vi "openCV_py.vi"() -> (2 "Move by":dbl[](array[numeric]))   [LabVIEW 2020]
panel:
  out "error out":errorcluster
  in  "error in (no error)":errorcluster
  in  "python module path":path=path "C:/Users/HEP/Documents/GitHub/UCSB-Gantry-HEP/Main VIs/LV_CV/py_cv.py"
  in  "python function name":string="get_new_loc"
  in  "Python version":string="3.6"
  out "PY time":dbl=1508.0
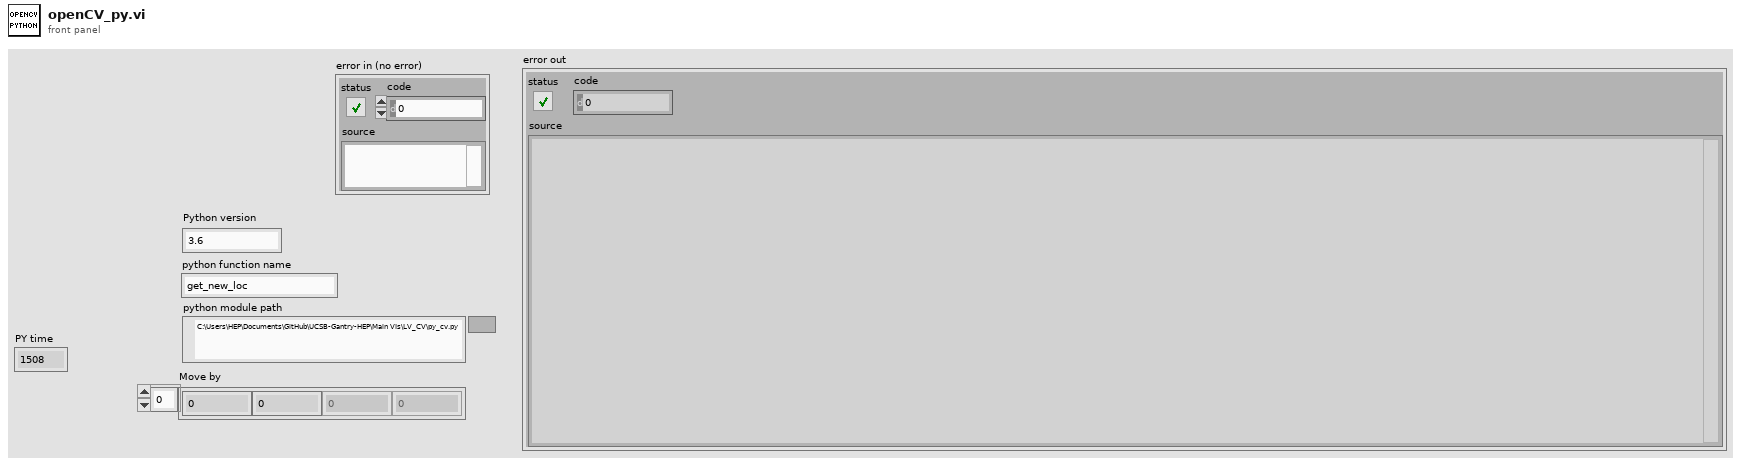
[diagram p1: front panel]
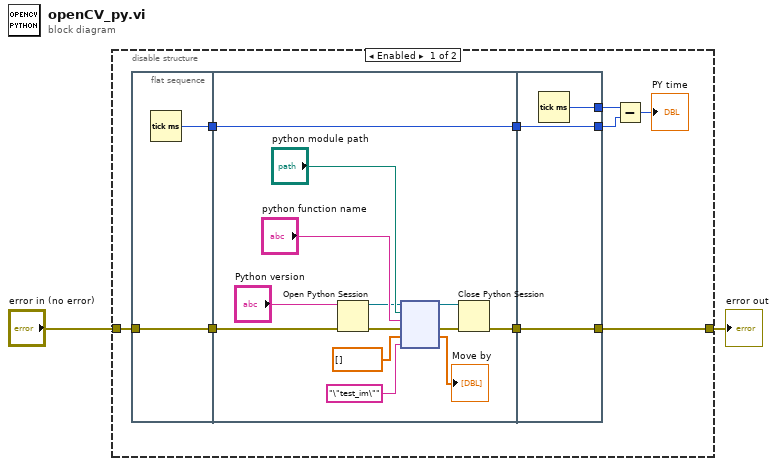
[diagram p0: block diagram]
diagram:
  n1 = disable-structure shown="Enabled" {
    disable-tunnel: "error in (no error)" -> [w7 _]
    disable-tunnel: [w6 _] -> w2
    frame Enabled {
      n2 = flat-sequence {
        tunnel: w7 -> [w13]
        tunnel: [w13] -> w11
        tunnel: [w12] -> w10
        tunnel: w11 -> [w21]
        tunnel: [w18] -> w9
        tunnel: [w17] -> w8
        tunnel: w10 -> [w17]
        tunnel: [w29] -> w6
        tunnel: w9 -> [w29]
        tunnel: [w28] -> w5
        tunnel: [w27] -> w4
        tunnel: w8 -> [w27]
        frame #0 {
          n3 = Tick Count (ms)() -> (millisecond timer value=w12:u32)
        }
        frame #1 {
          n4 = Open Python Session(python version="Python version", 3:w21) -> (session out=w23:refnum<k35>, error out=w20:errorcluster)  [unwired: 1 in]
          n5 = node(w23, "python module path", "python function name", w20, dbl[] [], "\"test_im\"") -> (w24:refnum<k35>, w19:errorcluster, →"Move by":dbl[])  [unwired: 1 in, 2 out]
          n6 = Close Python Session(session in=w24, error in=w19) -> (11:w18:errorcluster)
        }
        frame #2 {
          n7 = Tick Count (ms)() -> (millisecond timer value=w28:u32)
        }
      }
      n8 = Subtract(x=w5, y=w4) -> (x-y=→"PY time":u32)
    }
    frame Disabled {
    }
  }
  "error out" <- w2
